vi "FPGAData NightVision.vi"(0 "FPGA VI Reference In":refnum<k20>, 1 "SSG Breaker":bool, 3 "PV Breaker":bool, 5 "Gen West On/Off":bool, 9 "Gen East On/Off":bool, 11 "Error In":errorcluster, 12 "HVAC CMD":bool, 13 "PC CMD":bool, 14 "Real Time State":T1) -> (4 "SSG Data Out":T2 {"SSG Active Current" format="%2.1f"; "PV Reactive Power (L1)" format="%2.1f"; "PV Reactive Power (L2)" format="%2.1f"; "PV Total Reactive Power" format="%2.1f"; "Gen Reactive Power (L1)" format="%2.1f"; "Gen Reactive Power (L2)" format="%2.1f"; "Gen Total Reactive Power" format="%2.1f"; "SSG Reactive Power (L1)" format="%2.1f"; "SSG Reactive Power (L2)" format="%2.1f"; "SSG Total Reactive Power" format="%2.1f"; "PV Total Current" format="%2.1f"; "PV Total Voltage" format="%2.1f"; "PV Active Power (L1)" format="%2.1f"; "PV Active Power (L2)" format="%2.1f"; "PV App Power (L1)" format="%2.1f"; "PV App Power (L2)" format="%2.1f"; "PV Total Active Power" format="%2.1f"; "PV Total App Power" format="%2.1f"; "PV Arms (L1)" format="%2.1f"; "PV Arms (L2)" format="%2.1f"; "PV Vrms (L1)" format="%2.1f"; "PV Vrms (L2)" format="%2.1f"; "Gen Total Current" format="%2.1f"; "SSG Total Current" format="%2.1f"; "Gen Total Voltage" format="%2.1f"; "SSG Total Voltage" format="%2.1f"; "Gen Active Power (L1)" format="%2.1f"; "Gen Active Power (L2)" format="%2.1f"; "SSG Active Power (L1)" format="%2.1f"; "SSG Active Power (L2)" format="%2.1f"; "Gen App Power (L1)" format="%2.1f"; "Gen App Power (L2)" format="%2.1f"; "SSG App Power (L1)" format="%2.1f"; "SSG App Power (L2)" format="%2.1f"; "Gen Total Active Power" format="%2.1f"; "Gen Total App Power" format="%2.1f"; "Gen Arms (L1)" format="%2.1f"; "Gen Arms (L2)" format="%2.1f"; "Gen Vrms (L1)" format="%2.1f"; "Gen Vrms (L2)" format="%2.1f"; "SSG Total Active Power" format="%2.1f"; "SSG Total App Power" format="%2.1f"; "SSG Arms (L1)" format="%2.1f"; "SSG Arms (L2)" format="%2.1f"; "SSG Vrms (L1)" format="%2.1f"; "SSG Vrms (L2)" format="%2.1f"}, 6 "Automatic Start":bool, 10 "HVAC FB":bool, 15 "Error Out":errorcluster)   [LabVIEW 2014]
uses:
  Controls/FPGA Data.ctl
  Controls/RT State.ctl
  <vilib>/Utility/error.llb/Error Cluster From Error Code.vi
  <vilib>/rvi/errors/niLvFpgaAdjustHostInterfaceError.vi
  <vilib>/rvi/interface/nirviReadWriteControl/nirviReadWriteControl.xnode
  NiFpgaLv.dll
  <vilib>/rvi/interface/Simulation/niFpgaSimulationCallBeginRW.vi
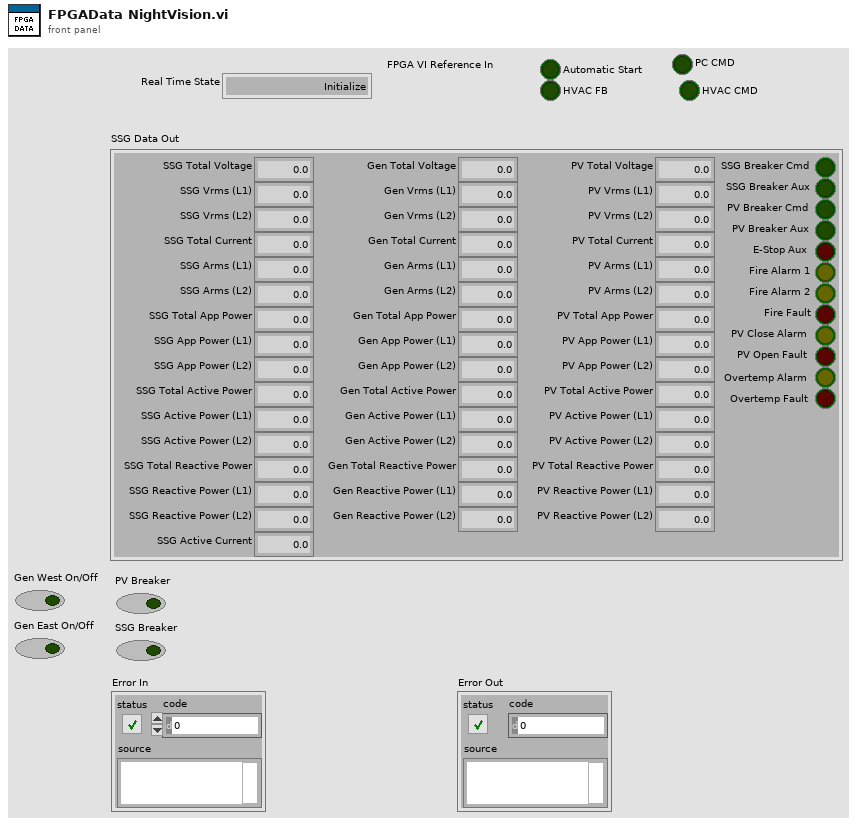
[diagram p1: front panel]
types:
  T1 = typedef "RT State.ctl" = enum16{"Initialize", "Ready", "Startup 1 - Start Genset", "Startup 2 - Start Inverter", "Startup 3 - Battery Match", "SpotGen - Start", "SpotGen - Charge", "SpotGen - Desync", "SpotGen - Discharge", "SpotGen - Sync", "Shutdown", "INVALID STATE"}
  T2 = typedef "FPGA Data.ctl" = cluster{"Gen Total Voltage":dbl, "Gen Vrms (L1)":dbl, "Gen Vrms (L2)":dbl, "Gen Total Current":dbl, "Gen Arms (L1)":dbl, "Gen Arms (L2)":dbl, "Gen Total App Power":dbl, "Gen App Power (L1)":dbl, "Gen App Power (L2)":dbl, "Gen Total Active Power":dbl, "Gen Active Power (L1)":dbl, "Gen Active Power (L2)":dbl, "Gen Total Reactive Power":dbl, "Gen Reactive Power (L1)":dbl, "Gen Reactive Power (L2)":dbl, "SSG Total Voltage":dbl, "SSG Vrms (L1)":dbl, "SSG Vrms (L2)":dbl, "SSG Total Current":dbl, "SSG Arms (L1)":dbl, "SSG Arms (L2)":dbl, "SSG Total App Power":dbl, "SSG App Power (L1)":dbl, "SSG App Power (L2)":dbl, "SSG Total Active Power":dbl, "SSG Active Power (L1)":dbl, "SSG Active Power (L2)":dbl, "SSG Total Reactive Power":dbl, "SSG Reactive Power (L1)":dbl, "SSG Reactive Power (L2)":dbl, "PV Total Voltage":dbl, "PV Vrms (L1)":dbl, "PV Vrms (L2)":dbl, "PV Total Current":dbl, "PV Arms (L1)":dbl, "PV Arms (L2)":dbl, "PV Total App Power":dbl, "PV App Power (L1)":dbl, "PV App Power (L2)":dbl, "PV Total Active Power":dbl, "PV Active Power (L1)":dbl, "PV Active Power (L2)":dbl, "PV Total Reactive Power":dbl, "PV Reactive Power (L1)":dbl, "PV Reactive Power (L2)":dbl, "SSG Breaker Cmd":bool, "SSG Breaker Aux":bool, "PV Breaker Cmd":bool, "PV Breaker Aux":bool, "E-Stop Aux":bool, "Fire Alarm 1":bool, "Fire Alarm 2":bool, "Fire Fault":bool, "PV Close Alarm":bool, "SSG Active Current":dbl, "Overtemp Alarm":bool, "Overtemp Fault":bool, "PV Open Fault":bool}
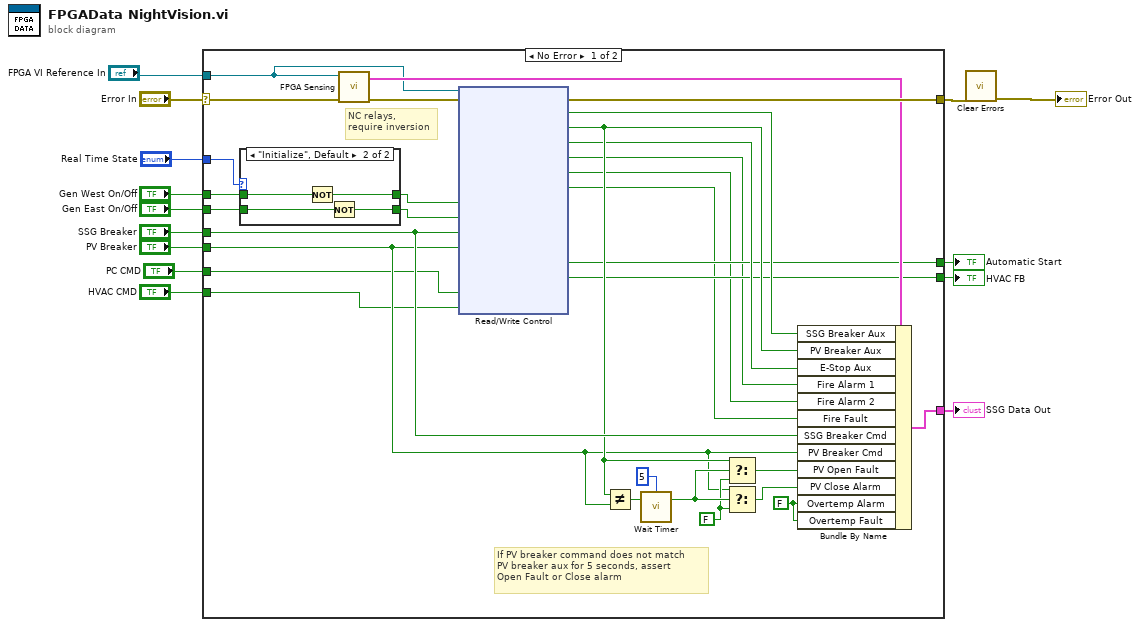
[diagram p0: block diagram]
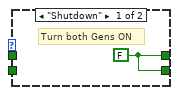
[diagram p2: hidden frame]
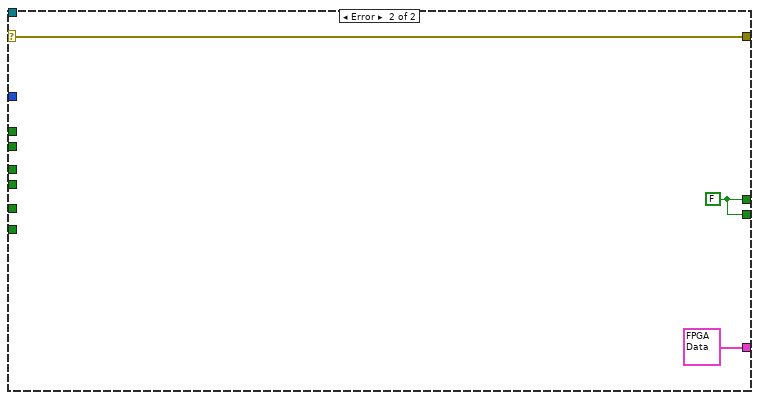
[diagram p3: hidden frame]
diagram:
  n1 = case shown="No Error" "Error In" {
    selector: "Error In" -> [w44 w52]
    tunnel: "FPGA VI Reference In" -> [w15 _]
    tunnel: [w42 w52] -> w2
    tunnel: [w41 T2 {"Gen Total Voltage"=0.0, "Gen Vrms (L1)"=0.0, "Gen Vrms (L2)"=0.0, "Gen Total Current"=0.0, "Gen Arms (L1)"=0.0, "Gen Arms (L2)"=0.0, "Gen Total App Power"=0.0, "Gen App Power (L1)"=0.0, "Gen App Power (L2)"=0.0, "Gen Total Active Power"=0.0, "Gen Active Power (L1)"=0.0, "Gen Active Power (L2)"=0.0, "Gen Total Reactive Power"=0.0, "Gen Reactive Power (L1)"=0.0, "Gen Reactive Power (L2)"=0.0, "SSG Total Voltage"=0.0, "SSG Vrms (L1)"=0.0, "SSG Vrms (L2)"=0.0, "SSG Total Current"=0.0, "SSG Arms (L1)"=0.0, "SSG Arms (L2)"=0.0, "SSG Total App Power"=0.0, "SSG App Power (L1)"=0.0, "SSG App Power (L2)"=0.0, "SSG Total Active Power"=0.0, "SSG Active Power (L1)"=0.0, "SSG Active Power (L2)"=0.0, "SSG Total Reactive Power"=0.0, "SSG Reactive Power (L1)"=0.0, "SSG Reactive Power (L2)"=0.0, "PV Total Voltage"=0.0, "PV Vrms (L1)"=0.0, "PV Vrms (L2)"=0.0, "PV Total Current"=0.0, "PV Arms (L1)"=0.0, "PV Arms (L2)"=0.0, "PV Total App Power"=0.0, "PV App Power (L1)"=0.0, "PV App Power (L2)"=0.0, "PV Total Active Power"=0.0, "PV Active Power (L1)"=0.0, "PV Active Power (L2)"=0.0, "PV Total Reactive Power"=0.0, "PV Reactive Power (L1)"=0.0, "PV Reactive Power (L2)"=0.0, "SSG Breaker Cmd"=FALSE, "SSG Breaker Aux"=FALSE, "PV Breaker Cmd"=FALSE, "PV Breaker Aux"=FALSE, "E-Stop Aux"=FALSE, "Fire Alarm 1"=FALSE, "Fire Alarm 2"=FALSE, "Fire Fault"=FALSE, "PV Close Alarm"=FALSE, "SSG Active Current"=0.0, "Overtemp Alarm"=FALSE, "Overtemp Fault"=FALSE, "PV Open Fault"=FALSE} ("SSG Data Out")] -> w13
    tunnel: "SSG Breaker" -> [w39 _]
    tunnel: "PV Breaker" -> [w31 _]
    tunnel: "Gen East On/Off" -> [w30 _]
    tunnel: "Gen West On/Off" -> [w29 _]
    tunnel: [w24 w50] -> w8
    tunnel: "HVAC CMD" -> [w23 _]
    tunnel: [w22 w50] -> w5
    tunnel: "Real Time State" -> [w17 _]
    tunnel: "PC CMD" -> [w16 _]
    frame No Error {
      w21 = FALSE ("Overtemp Alarm")
      w35 = FALSE
      # "NC relays, \nrequire inversion"
      # "If PV breaker command does not match\nPV breaker aux for 5 seconds, assert\nOpen Fault or Close alarm"
      n2 = case shown="\"Initialize\", Default" w17 {
        tunnel: w30 -> [_ w49]
        tunnel: w29 -> [_ w48]
        tunnel: [w45 w47] -> w28
        tunnel: [w45 w46] -> w27
        frame "Shutdown" {
          w45 = FALSE
          # "Turn both Gens ON"
        }
        frame "Initialize", Default {
          n3 = Not(x=w48) -> (.not. x?=w47:bool)
          n4 = Not(x=w49) -> (.not. x?=w46:bool)
        }
      }
      n5 = call "FPGA Sensing.vi"("Error In"=w44, "FPGA VI Reference In"=w15) -> ("Error Out"=w43:errorcluster, "SSG Data Out"=w26:T2)  [unwired: 8 in]
      n6 = xnode "Read/Write Control"("FPGA VI Reference In"=w15, "error in"=w43, "Gen West On/Off"=w28, "Gen East On/Off"=w27, "SSG Bkr"=w39, "PV Bkr"=w31, "PC CMD"=w16, "HVAC CMD"=w23) -> ("error out"=w42:errorcluster, "SSG Bkr Aux"=w40:bool, "PV Bkr Aux"=w32:bool, "E-Stop Aux"=w25:bool, "Fire Alarm 1"=w19:bool, "Fire Alarm 2"=w18:bool, "Fire Fault"=w20:bool, "AutoSwitch FB"=w24:bool, "HVAC FB"=w22:bool)  [unwired: 1 out]
      n7 = Not Equal?(x=w32, y=w31) -> (x != y?=w38:bool)
      n8 = call "Wait Timer.vi"("Boolean In"=w38, "Timer"=u32 5) -> ("Boolean Out"=w36:bool)  [unwired: 3 in]
      n9 = Select(t=w32, s=w36, f=w35) -> (s? t:f=w34:bool)
      n10 = Select(t=w31, s=w36, f=w35) -> (s? t:f=w33:bool)
      n11 = Bundle By Name(cluster=w26, "SSG Breaker Aux"=w40, "PV Breaker Aux"=w32, "E-Stop Aux"=w25, "Fire Alarm 1"=w19, "Fire Alarm 2"=w18, "Fire Fault"=w20, "SSG Breaker Cmd"=w39, "PV Breaker Cmd"=w31, "PV Open Fault"=w34, "PV Close Alarm"=w33, "Overtemp Alarm"=w21, "Overtemp Fault"=w21) -> (w41:T2)
    }
    frame Error {
      w50 = FALSE
    }
  }
  "SSG Data Out" <- w13
  "Automatic Start" <- w8
  "HVAC FB" <- w5
  n12 = call <vilib>:"Clear Errors.vi"("error in (no error)"=w2) -> ("error out"=→"Error Out":errorcluster)  [unwired: 5 in, 1 out]
